vi "Single plant data.vi"(0 "binarypath":path=path "J:/2017-5-18/2017-5-18-1/2017-5-18-1Rename/binary/C001-1", 1 "waveLengthNumber":i32=250, 2 "waveLengthSample":i32=1004, 5 "whitepath":path=path "J:/2017-5-18/2017-5-18-1/20170518075029whiteboard", 9 "blackpath":path=path "J:/2017-5-18/2017-5-18-1/20170518074900Black", 11 "imagepath":path=path "J:/2017-5-18/2017-5-18-1/2017-5-18-1Rename/result/C001-1.png", 12 "imageWidth":i32=700) -> (4 "output":dbl[](array[numeric]))   [LabVIEW 2015]
uses:
  <vilib>/vision/NI_Vision_Development_Module.lvlib
  Dll/HyperImageBinarization.dll
panel:
  out "Image":T1(plugin-control)
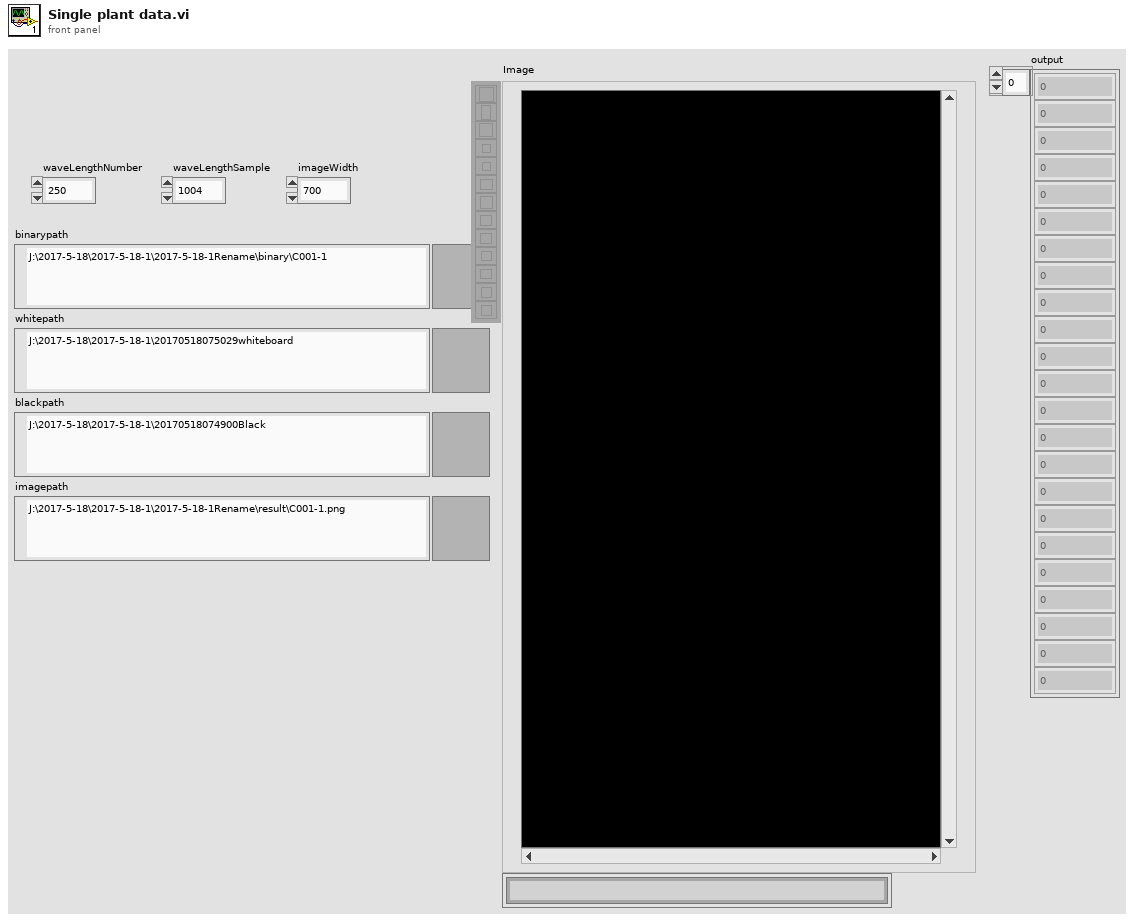
[diagram p1: front panel]
types:
  T1 = typedef "IMAQ Image.ctl" = refnum<image>
  T2 = enum32{"AutoM", "Close", "Dilate", "Erode", "Gradient", "Gradient out", "Gradient in", "Hit miss", "Open", "PClose", "POpen", "Thick", "Thin"}
  T3 = typedef "Image Type" = u32
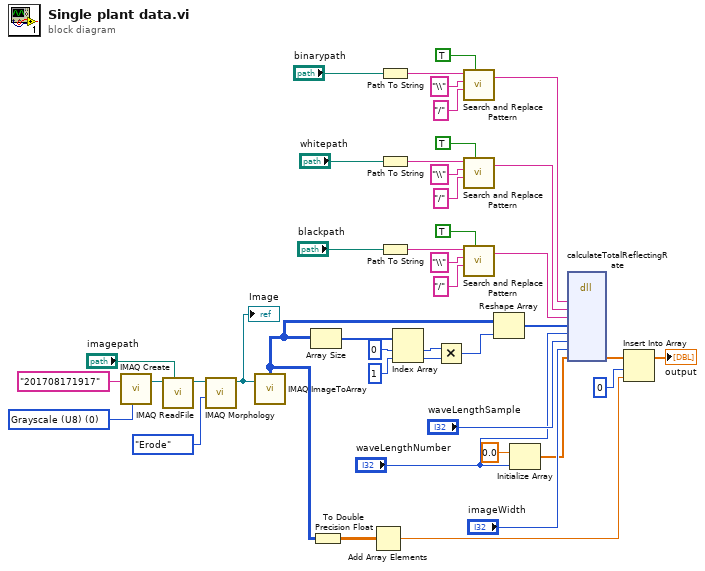
[diagram p0: block diagram]
diagram:
  w22 = T3 0 items=["Grayscale (U8)", "Grayscale (I16)", "Grayscale (SGL)", "Complex (CSG)", "RGB (U32)", "HSL (U32)", "RGB (U64)", "Grayscale (U16)"] ("Image Type")
  n1 = call "IMAQ Create"("Image Name"="201708171917", "Image Type"=w22) -> ("New Image"=w24:T1)  [unwired: 3 in, 1 out]
  n2 = call "IMAQ ReadFile"("File Path"="imagepath", "Image"=w24) -> ("Image Out"=w9:T1)  [unwired: 5 in, 4 out]
  n3 = call "IMAQ Morphology"("Operation"=T2."Erode", "Image Src"=w9) -> ("Image Dst Out"=w7:T1)  [unwired: 8 in, 1 out]
  "Image" <- w7
  n4 = call "IMAQ ImageToArray"("Image"=w7) -> ("Image Pixels (U8)"=w6:u8[][])  [unwired: 3 in, 4 out]
  n5 = Array Size(array=w6) -> (size(s)=w21:i32[])
  n6 = To Double Precision Float(number=w6) -> (double precision float=w5:dbl[][])
  n7 = Add Array Elements(numeric array=w5) -> (sum=w2:dbl)
  n8 = Path To String(path="binarypath") -> (string=w43:string)
  n9 = Path To String(path="whitepath") -> (string=w34:string)
  n10 = Path To String(path="blackpath") -> (string=w33:string)
  n11 = Index Array(array=w21, index #1=0 ("index"), index #2=1 ("index")) -> (element #1=w18:i32, element #2=w17:i32)
  n12 = Multiply(x=w18, y=w17) -> (x*y=w16:i32)
  n13 = call <vilib>:"Search and Replace Pattern.vi"("string"=w43, "regular expression (\"\")"="\\" ("regular expression (\"\")"), "replace string (\"\")"="/" ("replace string (\"\")"), "replace all? (F)"=TRUE) -> ("result string"=w28:string)  [unwired: 2 out]
  n14 = call <vilib>:"Search and Replace Pattern.vi"("string"=w34, "regular expression (\"\")"="\\" ("regular expression (\"\")"), "replace string (\"\")"="/" ("replace string (\"\")"), "replace all? (F)"=TRUE) -> ("result string"=w27:string)  [unwired: 2 out]
  n15 = call <vilib>:"Search and Replace Pattern.vi"("string"=w33, "regular expression (\"\")"="\\" ("regular expression (\"\")"), "replace string (\"\")"="/" ("replace string (\"\")"), "replace all? (F)"=TRUE) -> ("result string"=w26:string)  [unwired: 2 out]
  n16 = Reshape Array(w6, w16) -> (w15:u8[])
  n17 = Initialize Array(0.0 ("element"), "waveLengthNumber") -> (w10:dbl[])
  n18 = dll-call lib="I:/2017 Maize-Hyper-Program/Dll/HyperImageBinarization.dll" fn="calculateTotalReflectingRate"("binarypath"=w28, "whitepath"=w27, "blackpath"=w26, "image"=w15, "waveLengthNumber"="waveLengthNumber", "waveLengthSample"="waveLengthSample", "imageWidth"="imageWidth", "output"=w10) -> ("output"=w4:dbl[])  [unwired: 11 in, 2 out]
  n19 = Insert Into Array(array=w4, index=0, new element=w2) -> (→"output":dbl[])
